vi "GetXYLocal.vi"(6 "VI with 3D Control":refnum<vi>, 8 "error in (no error)":errorcluster, 10 "Global Mouse Coords":T1, 11 "Control Window in":refnum<class "Control Window.lvclass">) -> (0 "error out":errorcluster, 2 "Local Mouse Coords":T1, 3 "Control Window out":refnum<class "Control Window.lvclass">)   [LabVIEW 2015, in "Control Window.lvclass"]
uses:
  Control Window.lvclass
  3D Scene/Mouse Coords.ctl
  Control Window.lvclass/Control Window.ctl
  Input/Input.lvclass
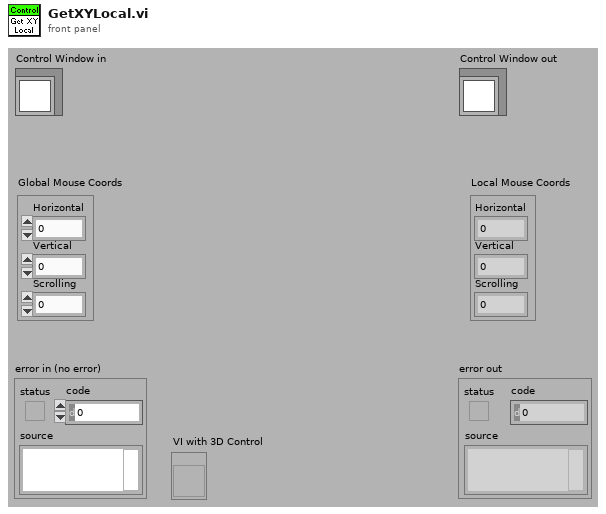
[diagram p1: front panel]
types:
  T1 = typedef "Input.lvclass/Mouse Coords.ctl" = cluster{"Horizontal":i32, "Vertical":i32, "Scrolling":i32}
  T2 = typedef "LVRectTypeDef.ctl" = cluster{"Left":i16, "Top":i16, "Right":i16, "Bottom":i16}
  T3 = typedef "LVPoint32TypeDef.ctl" = cluster{"Horizontal":i32, "Vertical":i32}
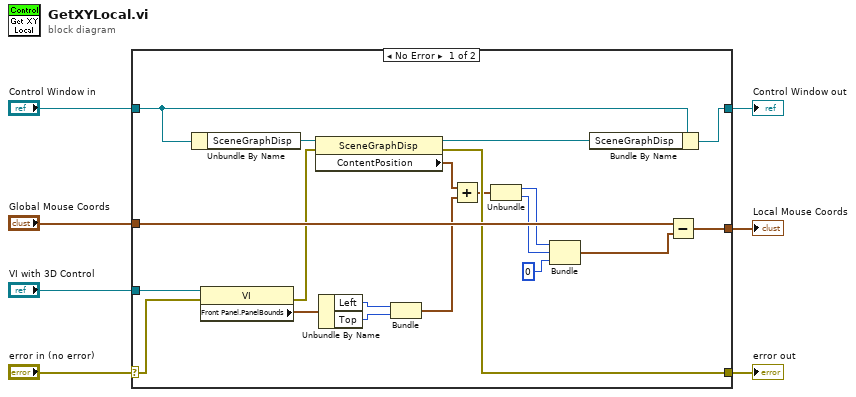
[diagram p0: block diagram]
diagram:
  n1 = case shown="No Error" "error in (no error)" {
    selector: "error in (no error)" -> [w15 w29]
    tunnel: [w13 w29] -> w6
    tunnel: [w23 w28] -> w4
    tunnel: "Control Window in" -> [w24 w28]
    tunnel: "Global Mouse Coords" -> [w26 _]
    tunnel: [w25 _] -> w1
    tunnel: "VI with 3D Control" -> [w21 _]
    frame No Error {
      n2 = Unbundle By Name(w24) -> ("SceneGraphDisp"=w27:refnum<vi>)
      n3 = property class="VI"(reference=w21, error in=w15) -> (error out=w14:errorcluster, "Front Panel.PanelBounds"=w20:T2)  [unwired: 1 out]
      n4 = property class="SceneGraphDisp"(reference=w27, error in=w14) -> (reference out=w22:refnum<vi>, error out=w13:errorcluster, "ContentPosition"=w16:T3)
      n5 = Unbundle By Name(w20) -> ("Left"=w18:i16, "Top"=w19:i16)
      n6 = Bundle("Left"=w18, "Top"=w19) -> (w17:cluster{"Left":i16, "Top":i16})  [unwired: 1 out]
      n7 = Add(x=w16, y=w17) -> (x+y=w12:T3)
      n8 = Unbundle(w12) -> ("Horizontal"=w11:i32, "Vertical"=w10:i32)
      n9 = Bundle("Horizontal"=w11, "Vertical"=w10, 0) -> (w8:cluster{"Horizontal":i32, "Vertical":i32, i32})  [unwired: 1 out]
      n10 = Bundle By Name(cluster=w24, "SceneGraphDisp"=w22) -> (w23:refnum<class "Control Window.lvclass">)
      n11 = Subtract(x=w26, y=w8) -> (x-y=w25:T1)
    }
    frame Error {
    }
  }
  "error out" <- w6
  "Control Window out" <- w4
  "Local Mouse Coords" <- w1
